vi "Arc Length of Bezier Spline.vi"(10 "ctrl pts":cluster{"x":sgl, "y":sgl}[][](array[cluster]), 11 "position":sgl[][](array[numeric])) -> (0 "t scaled":sgl[][](array[numeric]), 1 "t":sgl[](array[numeric]), 2 "l total":dbl, 3 "l":dbl[](array[numeric]))   [LabVIEW 2025]
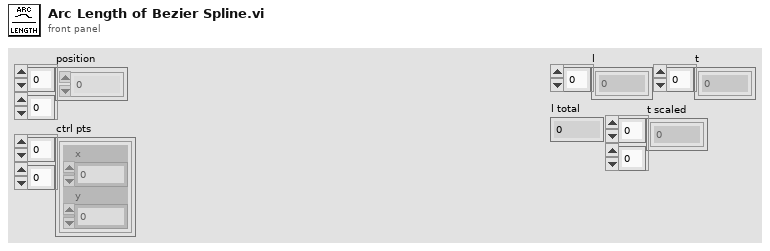
[diagram p1: front panel]
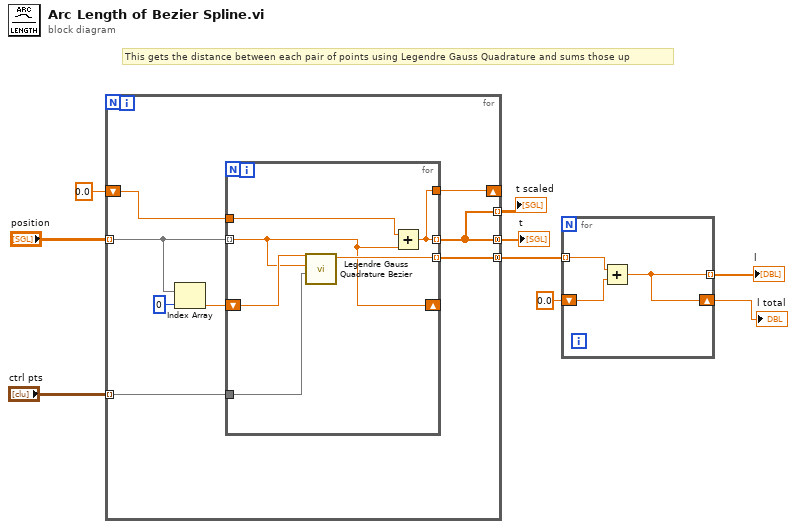
[diagram p0: block diagram]
diagram:
  # "This gets the distance between each pair of points using Legendre Gauss Quadrature and sums those up"
  n1 = for {
    tunnel: "position" -> [w16] mode=indexing
    tunnel: "ctrl pts" -> [w14] mode=indexing
    tunnel: [w13] -> w7 mode=concatenating
    tunnel: [w10] -> w2 mode=concatenating
    shift-right: [w11] -> _
    shift-left: sgl 0.0 ("percision") -> [w12]
    tunnel: [w10] -> w1 mode=indexing
    n2 = Index Array(array=w16, index=0) -> (element=w17:sgl)
    n3 = for {
      tunnel: w16 -> [w20] mode=indexing
      shift-right: [w20] -> _
      shift-left: w17 -> [w23]
      tunnel: w14 -> [w22]
      tunnel: [w21] -> w13 mode=indexing
      tunnel: [w18] -> w10 mode=indexing
      tunnel: w12 -> [w19]
      tunnel: [w18] -> w11
      n4 = call "Legendre Gauss Quadrature Bezier.vi"("ctrl points"=w22, "t1"=w20, "t0"=w23) -> ("l"=w21:dbl)  [unwired: 8 in]
      n5 = Add(x=w19, y=w20) -> (x+y=w18:sgl)
    }
  }
  "t" <- w2
  "t scaled" <- w1
  n6 = for {
    tunnel: w7 -> [w26] mode=indexing
    shift-right: [w24] -> w4
    shift-left: 0.0 ("l total") -> [w25]
    tunnel: [w24] -> w5 mode=indexing
    n7 = Add(x=w26, y=w25) -> (x+y=w24:dbl)
  }
  "l" <- w5
  "l total" <- w4
